vi "读取配置文件.vi"(8 "error in":errorcluster caption="错误输入（无错误）", 10 "配置":string(combo)) -> (0 "error out":errorcluster caption="错误输出", 2 "路径":string)   [LabVIEW 2020]
uses:
  <vilib>/Utility/config.llb/Read Key (String).vi
  <vilib>/Utility/config.llb/NI_LVConfig.lvlib
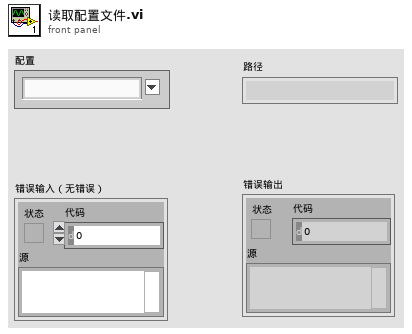
[diagram p1: front panel]
types:
  T1 = typedef "NI_LVConfig.lvlib/Config Data RefNum.ctl" = refnum<k1>
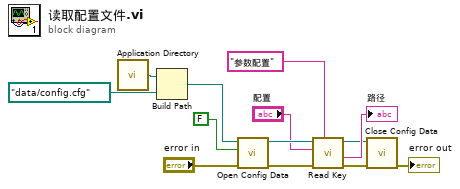
[diagram p0: block diagram]
diagram:
  n1 = call <vilib>:"Application Directory.vi"() -> ("Application Directory"=w13:path)
  n2 = Build Path(base path=w13, name or relative path=path "data/config.cfg") -> (appended path=w11:path)
  n3 = call <vilib>:"Open Config Data.vi"("error in (no error)"="error in", "create file if necessary (T)"=FALSE, "configuration file path"=w11) -> ("error out"=w7:errorcluster, "refnum"=w8:T1)  [unwired: 6 in, 1 out]
  n4 = call-poly <vilib>:"Read Key.vi"("section"="参数配置", "error in (no error)"=w7, "key"="配置", "refnum"=w8) -> ("error out"=w2:errorcluster, "value"=→"路径":string, "refnum out"=w3:T1)  [unwired: 4 in, 1 out]
  n5 = call <vilib>:"Close Config Data.vi"("error in (no error)"=w2, "refnum"=w3) -> ("error out"=→"error out":errorcluster)  [unwired: 8 in, 1 out]
